vi "Recebe serial.vi"(8 "error in (no error)":errorcluster, 11 "LNA VISA resource name":refnum<visa-resource-name>) -> (0 "error out":errorcluster, 1 "timeout":bool, 2 "String Lida":string, 3 "VISA Out":refnum<visa-resource-name>)   [LabVIEW 2018]
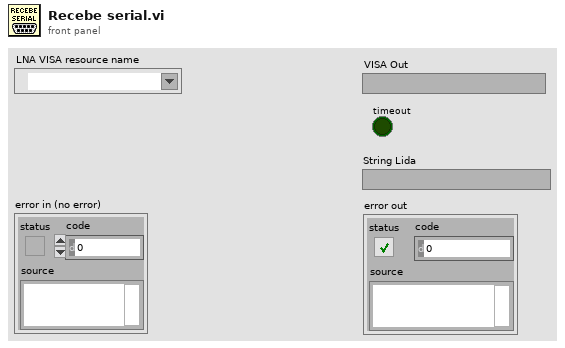
[diagram p1: front panel]
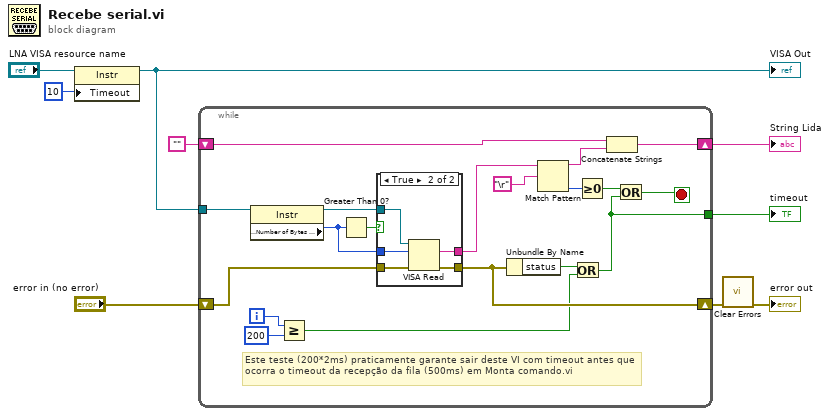
[diagram p0: block diagram]
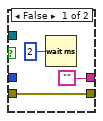
[diagram p2: hidden frame]
diagram:
  n1 = property class="Instr"(reference="LNA VISA resource name", "Timeout"=u32 10 ("General Settings:Timeout Value")) -> (reference out=w6:refnum<visa-resource-name>)  [unwired: 1 in, 1 out]
  "VISA Out" <- w6
  n2 = while {
    tunnel: w6 -> [w24]
    shift-right: [w27] -> w8
    shift-left: "" -> [w28]
    tunnel: [w16] -> w3
    shift-right: [w17] -> w2
    shift-left: "error in (no error)" -> [w26]
    i -> [w14]
    stop <- w25 stop-if-true
    # "Este teste (200*2ms) praticamente garante sair deste VI com timeout antes que ocorra o timeout da recepção da fila (500ms) em Monta comando.vi"
    n3 = property class="Instr"(reference=w24) -> (reference out=w23:refnum<visa-resource-name>, "Serial Settings:Number of Bytes at Serial Port"=w11:u32)  [unwired: 1 in, 1 out]
    n4 = Greater Or Equal?(x=w14, y=200) -> (x >= y?=w12:bool)
    n5 = Greater Than 0?(x=w11) -> (x > 0?=w10:bool)
    n6 = case shown="True" w10 {
      tunnel: w26 -> [w30 w36]
      tunnel: w23 -> [_ w35]
      tunnel: ["" w34] -> w22
      tunnel: [w30 w33] -> w17
      tunnel: w11 -> [_ w32]
      frame False {
        n7 = Wait (ms)(milliseconds to wait=u32 2) -> ()  [unwired: 1 out]
      }
      frame True {
        n8 = VISA Read(VISA resource name=w35, byte count=w32, error in (no error)=w36) -> (read buffer=w34:string, error out=w33:errorcluster)  [unwired: 2 out]
      }
    }
    n9 = Unbundle By Name(w17) -> ("status"=w15:bool)
    n10 = Match Pattern(string=w22, regular expression="\r") -> (before substring=w20:string, offset past match=w19:i32)  [unwired: 1 in, 2 out]
    n11 = Or(x=w15, y=w12) -> (x .or. y?=w16:bool)
    n12 = Greater Or Equal To 0?(x=w19) -> (x >= 0?=w18:bool)
    n13 = Concatenate Strings(w28, w20) -> (w27:string)
    n14 = Or(x=w18, y=w16) -> (x .or. y?=w25:bool)
  }
  "String Lida" <- w8
  "timeout" <- w3
  n15 = call <vilib>:"Clear Errors.vi"("error in (no error)"=w2) -> ("error out"=→"error out":errorcluster)  [unwired: 5 in, 1 out]
